vi "Reset encoder to slow speed_.vi"(8 "error in (no error)":errorcluster, 11 "Logging queue element":T1={"Imaging Protocol"=enum."Live Imaging", "Number of Trials"=0, "Frame Size"=512, "# Averaged frames"=0, "Dwell time (us)"=0.0, "Index of Z-plane"=0, "Timelapse?"=FALSE, "Logging process is active"=FALSE, "Speed logging enabled"=FALSE, "tdms file ref"=refnum, "path"=path "", "Trial Number"=0, "Expected # points acquired"=FALSE, "Manually stopped"=FALSE, "Last trial"=FALSE, "Ch0 data"=[], "Ch1 data"=[], "Ref Data"=[], "Ref Frame Time"=[], "Image Time"=[], "Continuous Time"=[], "Ref X Length"=0, "Ref Y Length"=0, "# Ref Averaged frames"=0, "Ref Dwell time (us)"=0.0, "Points acquired"={"Ch0 last trial"=0, "Ch1 last trial"=0, "All trials"=0}, "HW Timings File"=refnum} {"Ref Dwell time (us)" format="%#.6g"; "Frame Size" items=["100X100"=100, "128X128"=128, "200X200"=200, "256X256"=256, "512X512"=512, "1024x1024"=1024, "2048x2048"=2048]; "Dwell time (us)" format="%#.6g"}) -> (0 "error out":errorcluster)   [LabVIEW 2020]
uses:
  Typedefs/Logging queue element.ctl
  Typedefs/Imaging Protocols enum.ctl
  Typedefs/Frame Size.ctl
  Typedefs/Acquired points count.ctl
  Typedefs/Read Write Enum.ctl
  Global Variables/General Globals.vi
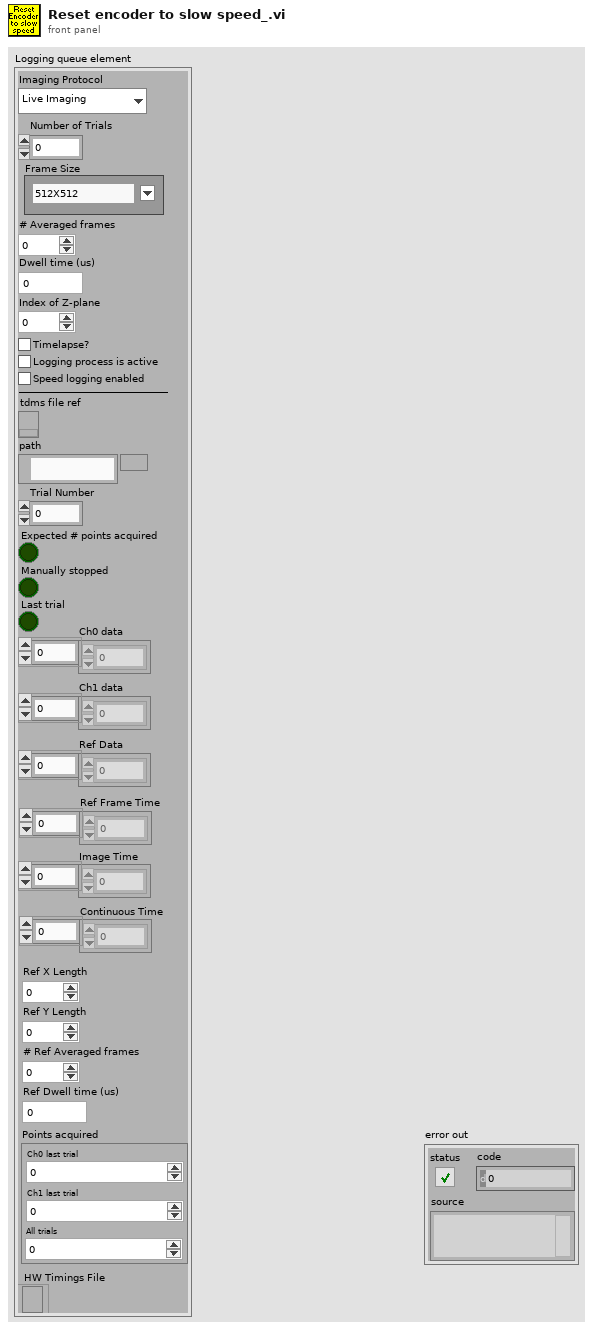
[diagram p1: front panel]
types:
  T1 = typedef "Logging queue element.ctl" = cluster{"Imaging Protocol":T2, "Number of Trials":u16, "Frame Size":T3, "# Averaged frames":u16, "Dwell time (us)":dbl, "Index of Z-plane":i32, "Timelapse?":bool, "Logging process is active":bool, "Speed logging enabled":bool, "tdms file ref":refnum<k34>, "path":path, "Trial Number":i32, "Expected # points acquired":bool, "Manually stopped":bool, "Last trial":bool, "Ch0 data":u32[], "Ch1 data":u32[], "Ref Data":u32[], "Ref Frame Time":u64[], "Image Time":u64[], "Continuous Time":u64[], "Ref X Length":u16, "Ref Y Length":u16, "# Ref Averaged frames":u16, "Ref Dwell time (us)":dbl, "Points acquired":T4, "HW Timings File":refnum<file>}
  T2 = typedef "Imaging Protocols enum.ctl" = enum16{"AOL Z-Stack", "Motor Z Stack", "Functional Acquisition", "Single Plane Acquisition", "Volume Acquisition", "Live Imaging", "Live Plane Imaging", "Live Volume Imaging"}
  T3 = typedef "Frame Size.ctl" = u16
  T4 = typedef "Acquired points count.ctl" = cluster{"Ch0 last trial":u64, "Ch1 last trial":u64, "All trials":u64}
  T5 = typedef "Read Write Enum.ctl" = enum16{"Read", "Write"}
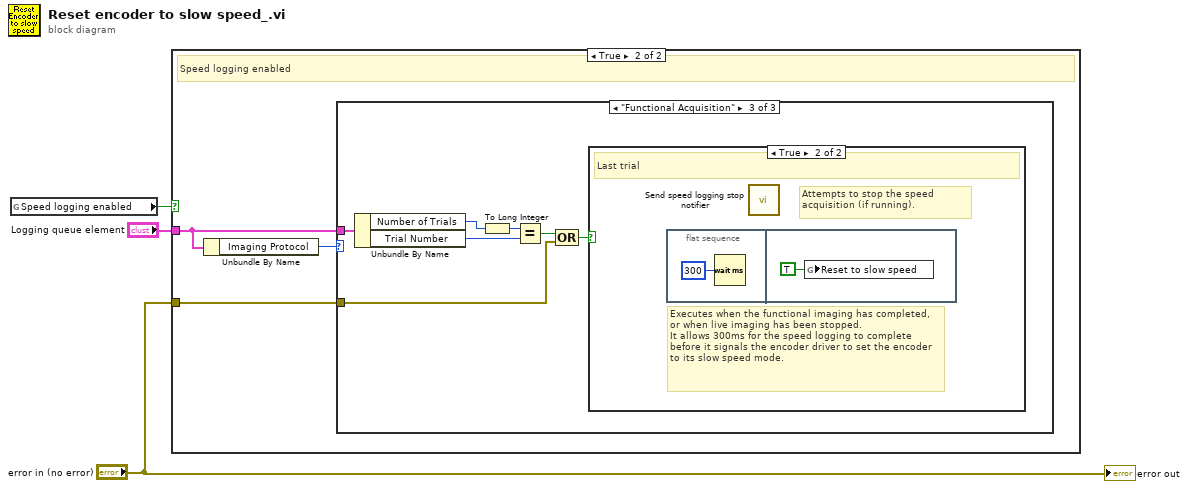
[diagram p0: block diagram]
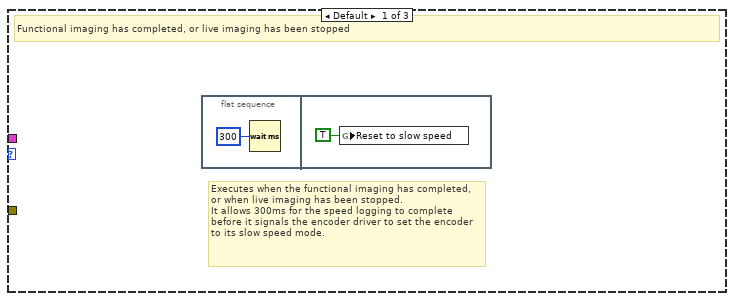
[diagram p3: hidden frame]
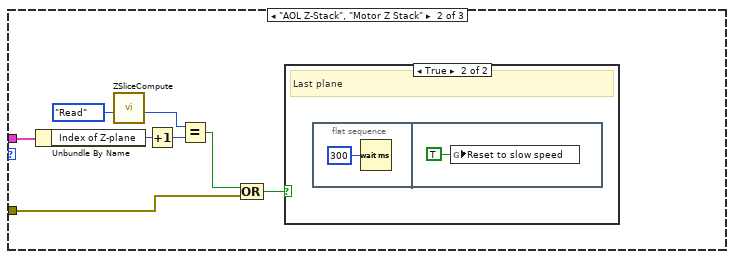
[diagram p4: hidden frame]
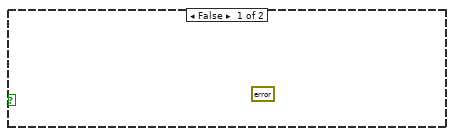
[diagram p6: hidden frame]
diagram:
  n1 = global read "General Globals.vi" "Speed logging enabled"() -> (w2:bool)
  n2 = case shown="True" w2 {
    tunnel: "Logging queue element" -> [_ w5]
    tunnel: "error in (no error)" -> [_ w4]
    frame False {
    }
    frame True {
      # "Speed logging enabled"
      n3 = Unbundle By Name(w5) -> ("Imaging Protocol"=w6:T2)
      n4 = case shown="\"Functional Acquisition\"" w6 {
        tunnel: w5 -> [_ w16 w20]
        tunnel: w4 -> [_ w11 w19]
        frame Default {
          # "Executes when the functional imaging has completed, or when live imaging has been stopped.\nIt allows 300ms for the speed logging to complete before it signals the encoder driver to set the encoder to its slow speed mode."
          # "Functional imaging has completed, or live imaging has been stopped"
          n5 = flat-sequence {
            frame #0 {
              n6 = Wait (ms)(milliseconds to wait=u32 300) -> ()  [unwired: 1 out]
            }
            frame #1 {
              n7 = global write "General Globals.vi" "Reset to slow speed"(TRUE ("Reset to slow speed")) -> ()
            }
          }
        }
        frame "AOL Z-Stack", "Motor Z Stack" {
          n8 = Unbundle By Name(w16) -> ("Index of Z-plane"=w15:i32)
          n9 = call "ZSliceCompute.vi"("Function"=Read_Write_Enum."Read") -> ("# of Z-planes"=w13:i32)  [unwired: 7 in, 3 out]
          n10 = Increment(x=w15) -> (x+1=w12:i32)
          n11 = Equal?(x=w13, y=w12) -> (x = y?=w10:bool)
          n12 = Compound Arithmetic op=OR(w10, w11) -> (w9:bool)
          n13 = case shown="True" w9 {
            frame False {
            }
            frame True {
              # "Last plane"
              n14 = flat-sequence {
                frame #0 {
                  n15 = Wait (ms)(milliseconds to wait=u32 300) -> ()  [unwired: 1 out]
                }
                frame #1 {
                  n16 = global write "General Globals.vi" "Reset to slow speed"(TRUE ("Reset to slow speed")) -> ()
                }
              }
            }
          }
        }
        frame "Functional Acquisition" {
          n17 = Unbundle By Name(w20) -> ("Number of Trials"=w24:u16, "Trial Number"=w25:i32)
          n18 = To Long Integer(number=w24) -> (32bit integer=w23:i32)
          n19 = Equal?(x=w23, y=w25) -> (x = y?=w22:bool)
          n20 = Compound Arithmetic op=OR(w22, w19) -> (w21:bool)
          n21 = case shown="True" w21 {
            frame False {
              (unwired) errorcluster {"status"=FALSE, "code"=0, "source"=""} ("error out (No error)")
            }
            frame True {
              # "Executes when the functional imaging has completed, or when live imaging has been stopped.\nIt allows 300ms for the speed logging to complete before it signals the encoder driver to set the encoder to its slow speed mode."
              # "Attempts to stop the speed acquisition (if running)."
              # "Last trial"
              n22 = flat-sequence {
                frame #0 {
                  n23 = Wait (ms)(milliseconds to wait=u32 300) -> ()  [unwired: 1 out]
                }
                frame #1 {
                  n24 = global write "General Globals.vi" "Reset to slow speed"(TRUE ("Reset to slow speed")) -> ()
                }
              }
              n25 = call "Send speed logging stop notifier.vi"() -> ()  [unwired: 11 in, 1 out]
            }
          }
        }
      }
    }
  }
  "error out" <- "error in (no error)"
